vi "GenerateTDMsFileName.vi"(10 "t0":timestamp, 11 "devime name":string) -> (2 "timestamp":timestamp, 3 "path":path)   [LabVIEW 2017, in "Tdms.lvlib"]
uses:
  <vilib>/addons/InsightCM/Utilities/Tdms/Tdms.lvlib
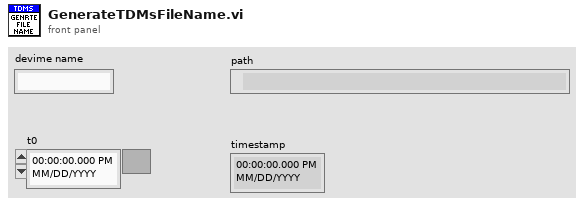
[diagram p1: front panel]
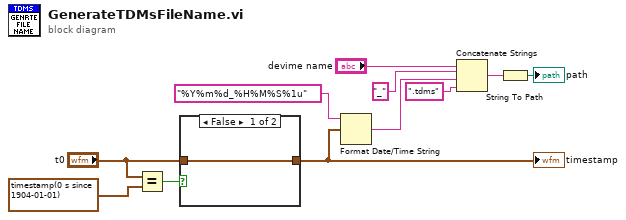
[diagram p0: block diagram]
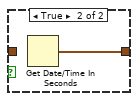
[diagram p2: hidden frame]
diagram:
  n1 = Equal?(x="t0", y=timestamp(0 s since 1904-01-01) ("t0")) -> (x = y?=w2:bool)
  n2 = case shown="False" w2 {
    tunnel: [w12 w13] -> w11
    tunnel: "t0" -> [w12 _]
    frame False {
    }
    frame True {
      n3 = Get Date/Time In Seconds() -> (seconds since 1Jan1904=w13:timestamp)
    }
  }
  "timestamp" <- w11
  n4 = Format Date/Time String(time format string (%c)="%Y%m%d_%H%M%S%1u", seconds (now)=w11) -> (date/time string=w7:string)  [unwired: 1 out]
  n5 = Concatenate Strings("devime name", "_" ("string"), w7, ".tdms" ("string")) -> (w9:string)
  n6 = String To Path(string=w9) -> (path=→"path":path)
